vi "Start test 2.vi"(8 "error in (no error)":errorcluster, 11 "Test_ExampleClassA in":refnum<class "Test_ExampleClassA.lvclass">) -> (0 "error out":errorcluster, 3 "Test_ExampleClassA out":refnum<class "Test_ExampleClassA.lvclass">)   [LabVIEW 2012, in "Test_ExampleClassA.lvclass"]
doc: "Starts subtest 2, which tests whether samples are properly produced by test subject."
uses:
  Test_ExampleClassA.lvclass
  Test settings cluster.ctl
  ExampleClassA/Settings cluster.ctl
  StartMessage/StartMessage.lvclass
  Test_ExampleClassA.lvclass/Test_ExampleClassA.ctl
  MurmexTest/MurmexTest.lvclass
  ExampleClassA/ExampleClassA.lvclass
  Murmex/Murmex.lvclass
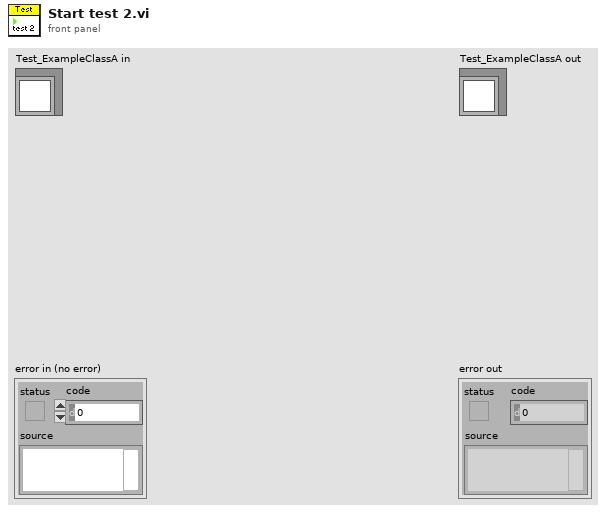
[diagram p1: front panel]
types:
  T1 = typedef "Test_ExampleClassA.lvclass/Test settings cluster.ctl" = cluster{"settings":T2, "valid?":bool}
  T2 = typedef "ExampleClassA.lvclass/Settings cluster.ctl" = cluster{"period?":dbl[unit], "number of blocks":i32, "number of channels":i32}
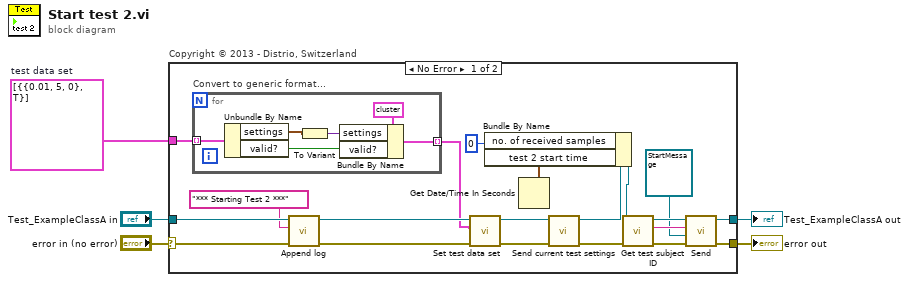
[diagram p0: block diagram]
diagram:
  w1 = T1[] [{"settings"={"period?"=0.01, "number of blocks"=5, "number of channels"=0}, "valid?"=TRUE}]  # test data set
  n1 = case "Copyright © 2013 - Distrio, Switzerland" shown="No Error" "error in (no error)" {
    selector: "error in (no error)" -> [w24 w33]
    tunnel: [w9 w33] -> w4
    tunnel: [w8 w32] -> w2
    tunnel: "Test_ExampleClassA in" -> [w23 w32]
    tunnel: w1 -> [w18 _]
    frame No Error {
      n2 = for "Convert to generic format..." {
        tunnel: w18 -> [w31] mode=indexing
        tunnel: [w26] -> w20 mode=indexing
        n3 = Unbundle By Name(w31) -> ("settings"=w27:T2, "valid?"=w29:bool)
        n4 = To Variant(anything=w27) -> (Variant=w28:variant)
        n5 = Bundle By Name(cluster=cluster{"settings":variant, "valid?":bool} {"settings"=variant, "valid?"=FALSE} ("test settings"), "settings"=w28, "valid?"=w29) -> (w26:cluster{"settings":variant, "valid?":bool})
      }
      n6 = call "Append log.vi"("error in (no error)"=w24, "log entry"="*** Starting Test 2 ***", "MurmexBase in"=w23) -> ("error out"=w19:errorcluster, "MurmexBase out"=w21:refnum<class "Test_ExampleClassA.lvclass">)  [unwired: 7 in]
      n7 = call "Set test data set.vi"("error in (no error)"=w19, "test settings"=w20, "MurmexTest in"=w21) -> ("error out"=w17:errorcluster, "MurmexTest out"=w13:refnum<class "Test_ExampleClassA.lvclass">)  [unwired: 7 in]
      n8 = Get Date/Time In Seconds() -> (seconds since 1Jan1904=w12:timestamp)
      n9 = call "Send current test settings.vi"("error in (no error)"=w17, "MurmexTest in"=w13) -> ("error out"=w16:errorcluster, "MurmexTest out"=w15:refnum<class "Test_ExampleClassA.lvclass">)  [unwired: 8 in]
      n10 = Bundle By Name(cluster=w15, "no. of received samples"=0 ("internal state.no. of received samples"), "test 2 start time"=w12) -> (w14:refnum<class "Test_ExampleClassA.lvclass">)
      n11 = call "Get test subject ID.vi"("error in (no error)"=w16, "MurmexTest in"=w14) -> ("error out"=w11:errorcluster, "test subject id"=w10:string, "MurmexTest out"=w7:refnum<class "Test_ExampleClassA.lvclass">)  [unwired: 7 in]
      n12 = call "Send.vi"("error in (no error)"=w11, "Message"=refnum<class "StartMessage.lvclass"> refnum ("StartMessage.lvclass"), "recipient"=w10, "Murmex in"=w7) -> ("error out"=w9:errorcluster, "Murmex out"=w8:refnum<class "Test_ExampleClassA.lvclass">)  [unwired: 6 in]
    }
    frame Error {
    }
  }
  "error out" <- w4
  "Test_ExampleClassA out" <- w2
